vi "WSVCAP SHL Host LL Remap DUT and Socket Locations.vi"(0 "C1 DUT Ordered Data In":u8[][](array[numeric]) format="%.0x", 1 "C2 DUT Ordered Data In":u8[][](array[numeric]) format="%.0x", 2 "C3 DUT Ordered Data In":u8[][](array[numeric]) format="%.0x", 3 "C1 Socket Ordered Data In":u8[][](array[numeric]) format="%.0x", 4 "C2 Socket Ordered Data In":u8[][](array[numeric]) format="%.0x", 5 "C3 Socket Ordered Data In":u8[][](array[numeric]) format="%.0x") -> (14 "C1 Socket Ordered Data Out":u8[][](array[numeric]) format="%.0x", 15 "C2 Socket Ordered Data Out":u8[][](array[numeric]) format="%.0x", 16 "C3 Socket Ordered Data Out":u8[][](array[numeric]) format="%.0x", 17 "C1 DUT Ordered Data Out":u8[][](array[numeric]) format="%.0x", 18 "C2 DUT Ordered Data Out":u8[][](array[numeric]) format="%.0x", 19 "C3 DUT Ordered Data Out":u8[][](array[numeric]) format="%.0x")   [LabVIEW 2012]
uses:
  Type Defs/WSVCAP SHL DUT Number Enum.ctl
panel:
  out "DUT/SOCKET Map":string[](array[string])=["DUT 01 [S08-H]", "DUT 02 [S07-G]", "DUT 03 [S09-I]", "DUT 04 [S10-J]", "DUT 05 [S06-F]", "DUT 06 [S05-E]", "DUT 07 [S12-L]", "DUT 08 [S11-K]", "DUT 09 [S03-C]", "DUT 10 [S04-D]", "DUT 11 [S13-M]", "DUT 12 [S14-N]", "DUT 13 [S02-B]", "DUT 14 [S01-A]", "DUT 15 [S16-P]", "DUT 16 [S15-O]"]
  in  "DUT Number":T1
  # "DUT 01"
  # "DUT 02"
  # "DUT 03"
  # "DUT 04"
  # "DUT 05"
  # "DUT 06"
  # "DUT 07"
  # "DUT 08"
  # "DUT 09"
  # "DUT 10"
  # "DUT 11"
  # "DUT 12"
  # "DUT 13"
  # "DUT 14"
  # "DUT 15"
  # "DUT 16"
  # "SKT 01"
  # "SKT 02"
  # "SKT 03"
  # "SKT 04"
  # "SKT 05"
  # "SKT 06"
  # "SKT 07"
  # "SKT 08"
  # "SKT 09"
  # "SKT 10"
  # "SKT 11"
  # "SKT 12"
  # "SKT 13"
  # "SKT 14"
  # "SKT 15"
  # "SKT 16"
  # "DUT 01"
  # "DUT 02"
  # "DUT 03"
  # "DUT 04"
  # "DUT 05"
  # "DUT 06"
  # "DUT 07"
  # "DUT 08"
  # "DUT 09"
  # "DUT 10"
  # "DUT 11"
  # "DUT 12"
  # "DUT 13"
  # "DUT 14"
  # "DUT 15"
  # "DUT 16"
  # "SKT 01"
  # "SKT 02"
  # "SKT 03"
  # "SKT 04"
  # "SKT 05"
  # "SKT 06"
  # "SKT 07"
  # "SKT 08"
  # "SKT 09"
  # "SKT 10"
  # "SKT 11"
  # "SKT 12"
  # "SKT 13"
  # "SKT 14"
  # "SKT 15"
  # "SKT 16"
  # "DUT 01"
  # "DUT 02"
  # "DUT 03"
  # "DUT 04"
  # "DUT 05"
  # "DUT 06"
  # "DUT 07"
  # "DUT 08"
  # "DUT 09"
  # "DUT 10"
  # "DUT 11"
  # "DUT 12"
  # "DUT 13"
  # "DUT 14"
  # "DUT 15"
  # "DUT 16"
  # "SKT 01"
  # "SKT 02"
  # "SKT 03"
  # "SKT 04"
  # "SKT 05"
  # "SKT 06"
  # "SKT 07"
  # "SKT 08"
  # "SKT 09"
  # "SKT 10"
  # "SKT 11"
  # "SKT 12"
  # "SKT 13"
  # "SKT 14"
  # "SKT 15"
  # "SKT 16"
  # "DUT 01"
  # "DUT 02"
  # "DUT 03"
  # "DUT 04"
  # "DUT 05"
  # "DUT 06"
  # "DUT 07"
  # "DUT 08"
  # "DUT 09"
  # "DUT 10"
  # "DUT 11"
  # "DUT 12"
  # "DUT 13"
  # "DUT 14"
  # "DUT 15"
  # "DUT 16"
  # "SKT 01"
  # "SKT 02"
  # "SKT 03"
  # "SKT 04"
  # "SKT 05"
  # "SKT 06"
  # "SKT 07"
  # "SKT 08"
  # "SKT 09"
  # "SKT 10"
  # "SKT 11"
  # "SKT 12"
  # "SKT 13"
  # "SKT 14"
  # "SKT 15"
  # "SKT 16"
  # "DUT 01"
  # "DUT 02"
  # "DUT 03"
  # "DUT 04"
  # "DUT 05"
  # "DUT 06"
  # "DUT 07"
  # "DUT 08"
  # "DUT 09"
  # "DUT 10"
  # "DUT 11"
  # "DUT 12"
  # "DUT 13"
  # "DUT 14"
  # "DUT 15"
  # "DUT 16"
  # "SKT 01"
  # "SKT 02"
  # "SKT 03"
  # "SKT 04"
  # "SKT 05"
  # "SKT 06"
  # "SKT 07"
  # "SKT 08"
  # "SKT 09"
  # "SKT 10"
  # "SKT 11"
  # "SKT 12"
  # "SKT 13"
  # "SKT 14"
  # "SKT 15"
  # "SKT 16"
  # "SKT 01"
  # "SKT 02"
  # "SKT 03"
  # "SKT 04"
  # "SKT 05"
  # "SKT 06"
  # "SKT 07"
  # "SKT 08"
  # "SKT 09"
  # "SKT 10"
  # "SKT 11"
  # "SKT 12"
  # "SKT 13"
  # "SKT 14"
  # "SKT 15"
  # "SKT 16"
  # "DUT 01"
  # "DUT 02"
  # "DUT 03"
  # "DUT 04"
  # "DUT 05"
  # "DUT 06"
  # "DUT 07"
  # "DUT 08"
  # "DUT 09"
  # "DUT 10"
  # "DUT 11"
  # "DUT 12"
  # "DUT 13"
  # "DUT 14"
  # "DUT 15"
  # "DUT 16"
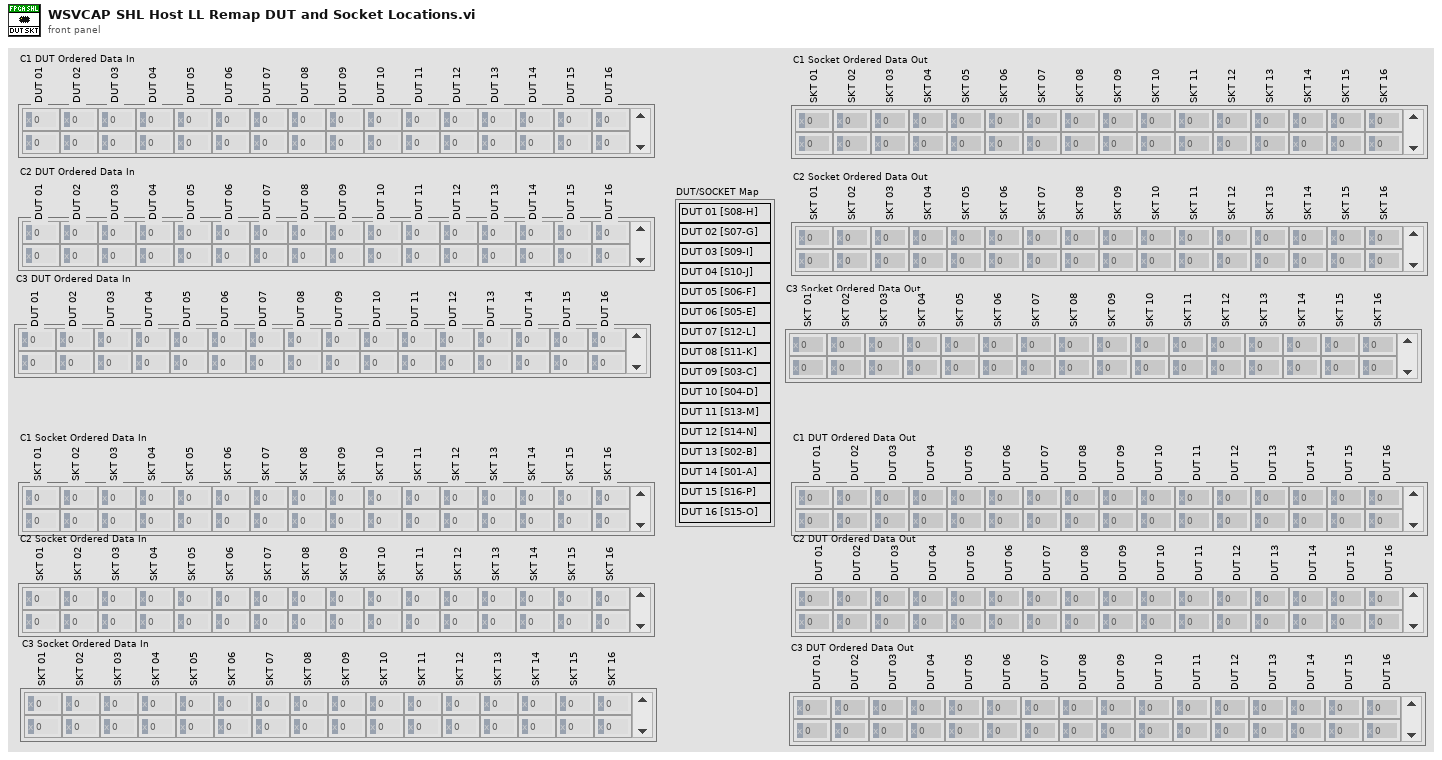
[diagram p1: front panel]
types:
  T1 = typedef "WSVCAP SHL DUT Number Enum.ctl" = enum16{"DUT 01", "DUT 02", "DUT 03", "DUT 04", "DUT 05", "DUT 06", "DUT 07", "DUT 08", "DUT 09", "DUT 10", "DUT 11", "DUT 12", "DUT 13", "DUT 14", "DUT 15", "DUT 16", "DUT 17", "DUT 18", "DUT 19", "DUT 20", "DUT 21", "DUT 22", "DUT 23", "DUT 24", "DUT 25", "DUT 26", "DUT 27", "DUT 28", "DUT 29", "DUT 30", "DUT 31", "DUT 32", "DUT 33", "DUT 34", "DUT 35", "DUT 36"}
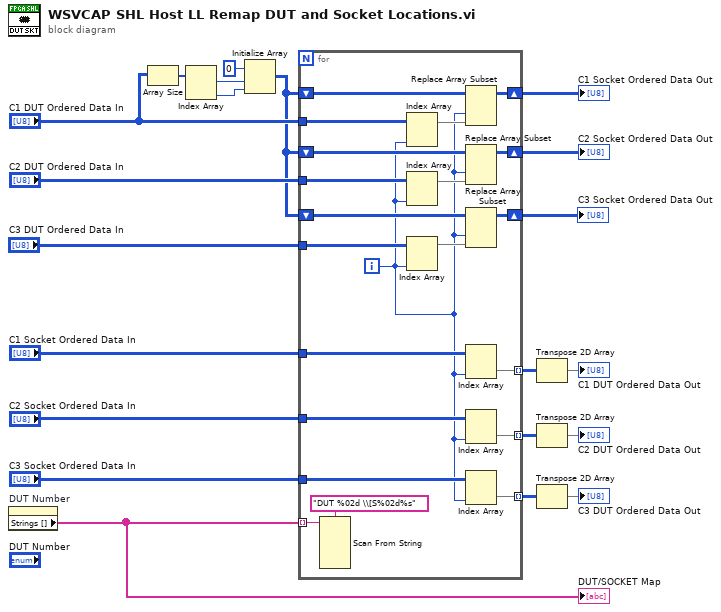
[diagram p0: block diagram]
diagram:
  n1 = property on="DUT Number" class="Enum (strict)"() -> ("Strings []"=w12:string[])  [unwired: 2 in, 2 out]
  "DUT/SOCKET Map" <- w12
  n2 = Array Size(array="C1 DUT Ordered Data In") -> (size(s)=w10:i32[])
  n3 = Index Array(array=w10) -> (element #1=w9:i32, element #2=w8:i32)  [unwired: 2 in]
  n4 = Initialize Array(u8 0 ("element"), w9, w8) -> (w5:u8[][])
  n5 = for {
    tunnel: w12 -> [w40] mode=indexing
    tunnel: "C1 DUT Ordered Data In" -> [w42]
    tunnel: "C1 Socket Ordered Data In" -> [w39]
    tunnel: [w38] -> w20 mode=indexing
    shift-right: [w36] -> w18
    shift-left: w5 -> [w37]
    shift-right: [w32] -> w16
    shift-left: w5 -> [w33]
    tunnel: "C2 DUT Ordered Data In" -> [w31]
    tunnel: "C2 Socket Ordered Data In" -> [w30]
    tunnel: [w29] -> w14 mode=indexing
    tunnel: "C3 DUT Ordered Data In" -> [w28]
    shift-right: [w26] -> w4
    shift-left: w5 -> [w27]
    tunnel: [w24] -> w3 mode=indexing
    tunnel: "C3 Socket Ordered Data In" -> [w23]
    i -> [w22]
    n6 = Scan From String(format string="DUT %02d \\[S%02d%s", input string=w40) -> ()  [unwired: 8 in, 3 out]
    n7 = Index Array(array=w42, index (col)=w22) -> (element=w35:u8[])  [unwired: 1 in]
    n8 = Index Array(array=w31, index (col)=w22) -> (element=w34:u8[])  [unwired: 1 in]
    n9 = Index Array(array=w28, index (col)=w22) -> (element=w25:u8[])  [unwired: 1 in]
    n10 = Replace Array Subset(array=w37, new element=w35, index (col)=w22) -> (w36:u8[][])  [unwired: 1 in]
    n11 = Replace Array Subset(array=w33, new element=w34, index (col)=w22) -> (w32:u8[][])  [unwired: 1 in]
    n12 = Replace Array Subset(array=w27, new element=w25, index (col)=w22) -> (w26:u8[][])  [unwired: 1 in]
    n13 = Index Array(array=w39, index (col)=w22) -> (element=w38:u8[])  [unwired: 1 in]
    n14 = Index Array(array=w30, index (col)=w22) -> (element=w29:u8[])  [unwired: 1 in]
    n15 = Index Array(array=w23, index (col)=w22) -> (element=w24:u8[])  [unwired: 1 in]
  }
  "C1 Socket Ordered Data Out" <- w18
  "C2 Socket Ordered Data Out" <- w16
  "C3 Socket Ordered Data Out" <- w4
  n16 = Transpose 2D Array(2D array=w20) -> (transposed array=→"C1 DUT Ordered Data Out":u8[][])
  n17 = Transpose 2D Array(2D array=w14) -> (transposed array=→"C2 DUT Ordered Data Out":u8[][])
  n18 = Transpose 2D Array(2D array=w3) -> (transposed array=→"C3 DUT Ordered Data Out":u8[][])
